vi "SW_Load_data_for_Analysis_from_TDMS.vi"(4 "Data samples to load":i64=-1, 6 "create index file? (T)":bool, 8 "error in (no error)":errorcluster, 9 "Progress bar reference":refnum<vi>, 10 "Cluster of paths input":T5, 11 "Data flow controls":T6) -> (0 "error out":errorcluster, 2 "Time to load, ms":u32, 3 "Loaded data":T1, 5 "Data loaded OK":bool, 7 "Settings loaded OK":bool)   [LabVIEW 2016]
panel:
  out "Loaded recording parameters":T2
  out "Author's name":string
  out "Stimulus presets array (loaded)":T3(array[cluster])
  out "Acquisition settings cluster out":T4
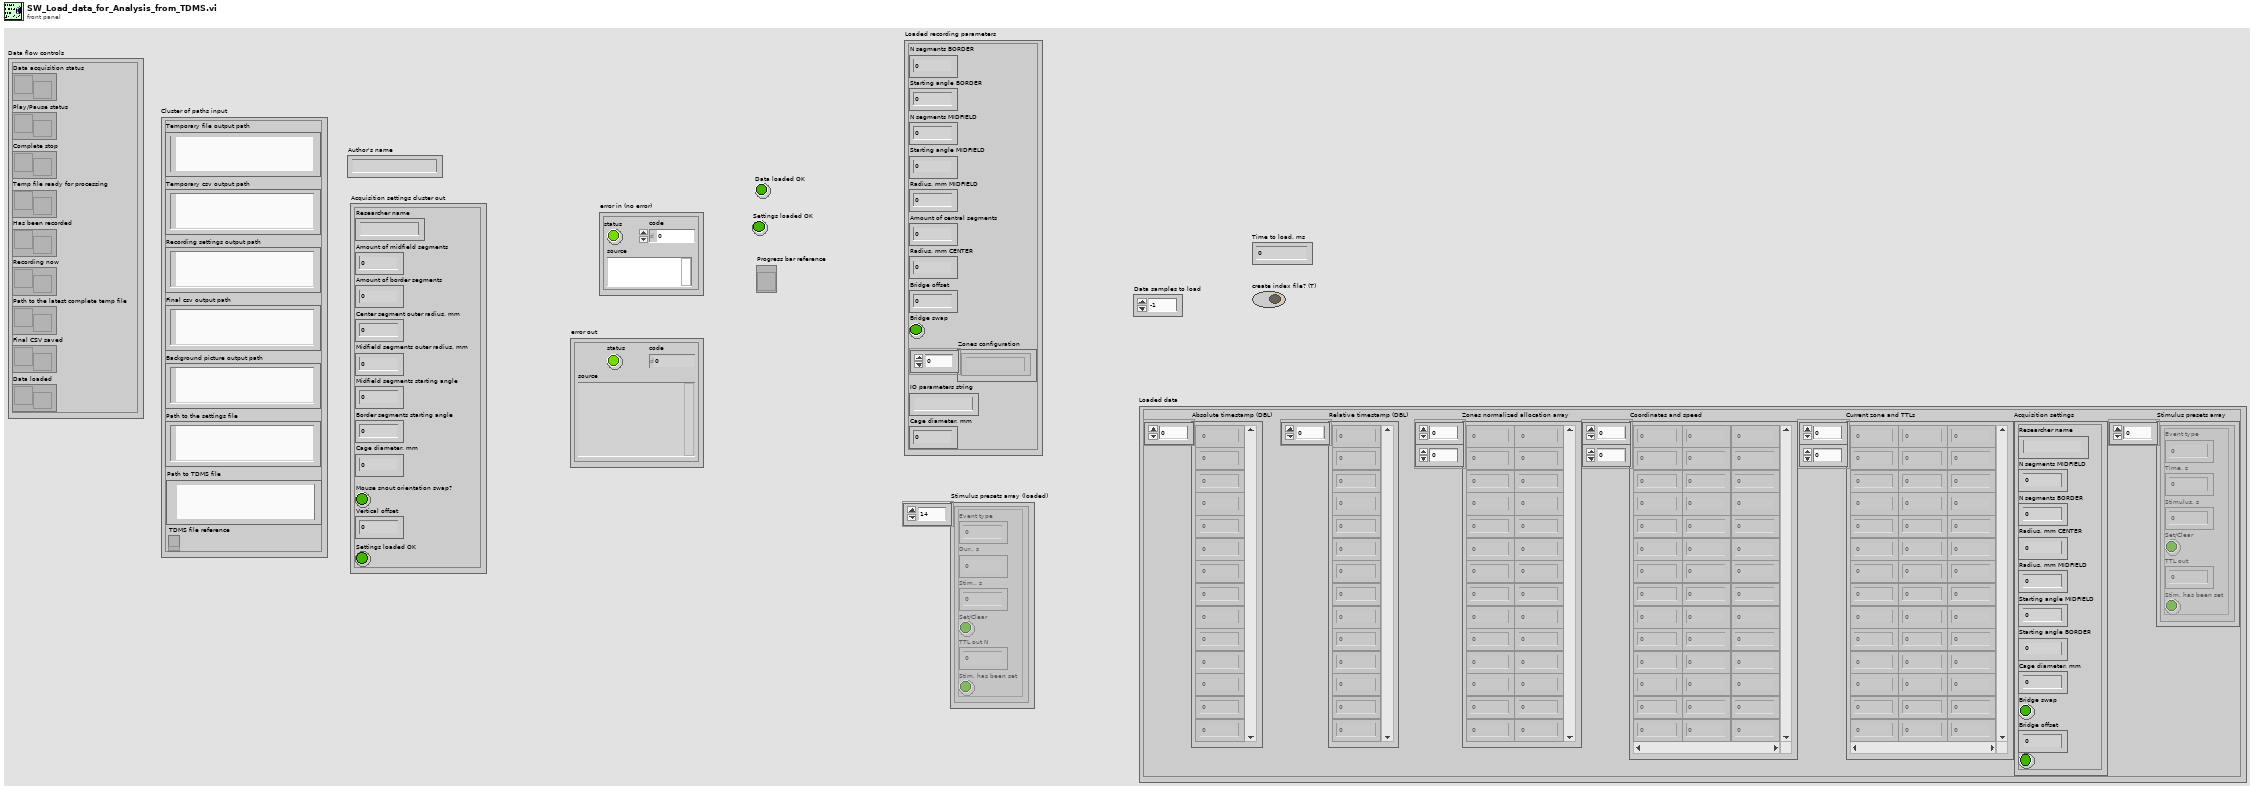
[diagram p1: front panel]
types:
  T1 = cluster{"Absolute timestamp (DBL)":dbl[], "Relative timestamp (DBL)":dbl[], "Zones normalized allocation array":dbl[][], "Coordinates and speed":dbl[][], "Current zone and TTLs":u8[][], "Acquisition settings":cluster{"Researcher name":string, "N segments MIDFIELD":u8, "N segments BORDER":u8, "Radius, mm CENTER":u16, "Radius, mm MIDFIELD":u16, "Starting angle MIDFIELD":i16, "Starting angle BORDER":i16, "Cage diameter, mm":u16, "Bridge swap":bool, "Bridge offset":sgl, "Boolean":bool}, "Stimulus presets array":cluster{"Event type":u16, "Time, s":sgl, "Stimulus, s":sgl, "Set/Clear":bool, "TTL out":u16, "Stim. has been set":bool}[]}
  T2 = cluster{"N segments BORDER":u8, "Starting angle BORDER":i16, "N segments MIDFIELD":u8, "Starting angle MIDFIELD":i16, "Radius, mm MIDFIELD":u16, "Amount of central segments":u8, "Radius, mm CENTER":u16, "Bridge offset":sgl, "Bridge swap":bool, "Zones configuration":string[], "IO parameters string":string, "Cage diameter, mm":u16}
  T3 = cluster{"Event type":u16, "Dur., s":sgl, "Stim., s":sgl, "Set/Clear":bool, "TTL out N":u16, "Stim. has been set":bool}[]
  T4 = cluster{"Researcher name":string, "Amount of midfield segments":u32, "Amount of border segments":u32, "Center segment outer radius, mm":u32, "Midfield segments outer radius, mm":u32, "Midfield segments starting angle":i32, "Border segments starting angle":i32, "Cage diameter, mm":u32, "Mouse snout orientation swap?":bool, "Vertical offset":dbl, "Settings loaded OK":bool}
  T5 = cluster{"Temporary file output path":path, "Temporary csv output path":path, "Recording settings output path":path, "Final csv output path":path, "Background picture output path":path, "Path to the settings file":path, "Path to TDMS file":path, "TDMS file reference":refnum<k34>}
  T6 = cluster{"Data acquisition status":refnum<notifier>, "Play/Pause status":refnum<notifier>, "Complete stop":refnum<notifier>, "Temp file ready for processing":refnum<notifier>, "Has been recorded":refnum<notifier>, "Recording now":refnum<notifier>, "Path to the latest complete temp file":refnum<notifier>, "Final CSV saved":refnum<notifier>, "Data loaded":refnum<notifier>}
  T7 = enum16{"big-endian, network order", "native, host order", "little-endian"}
  T8 = enum16{"open", "open or create", "create or replace", "create", "open (read-only)"}
  T9 = cluster{"Event type":u16, "Time, s":sgl, "Stimulus, s":sgl, "Set/Clear":bool, "TTL out":u16, "Stim. has been set":bool}
  T10 = cluster{string, "N segments MIDFIELD":u8, "N segments BORDER":u8, "Radius, mm CENTER":u16, "Radius, mm MIDFIELD":u16, "Starting angle MIDFIELD":i16, "Starting angle BORDER":i16, "Cage diameter, mm":u16, "Bridge swap":bool, "Bridge offset":sgl, bool}
  T11 = cluster{dbl[], dbl[], "Zones normalized allocation array":dbl[][], dbl[][], u8[][], cluster{string, "N segments MIDFIELD":u8, "N segments BORDER":u8, "Radius, mm CENTER":u16, "Radius, mm MIDFIELD":u16, "Starting angle MIDFIELD":i16, "Starting angle BORDER":i16, "Cage diameter, mm":u16, "Bridge swap":bool, "Bridge offset":sgl, bool}, cluster{"Event type":u16, "Time, s":sgl, "Stimulus, s":sgl, "Set/Clear":bool, "TTL out":u16, "Stim. has been set":bool}[]}
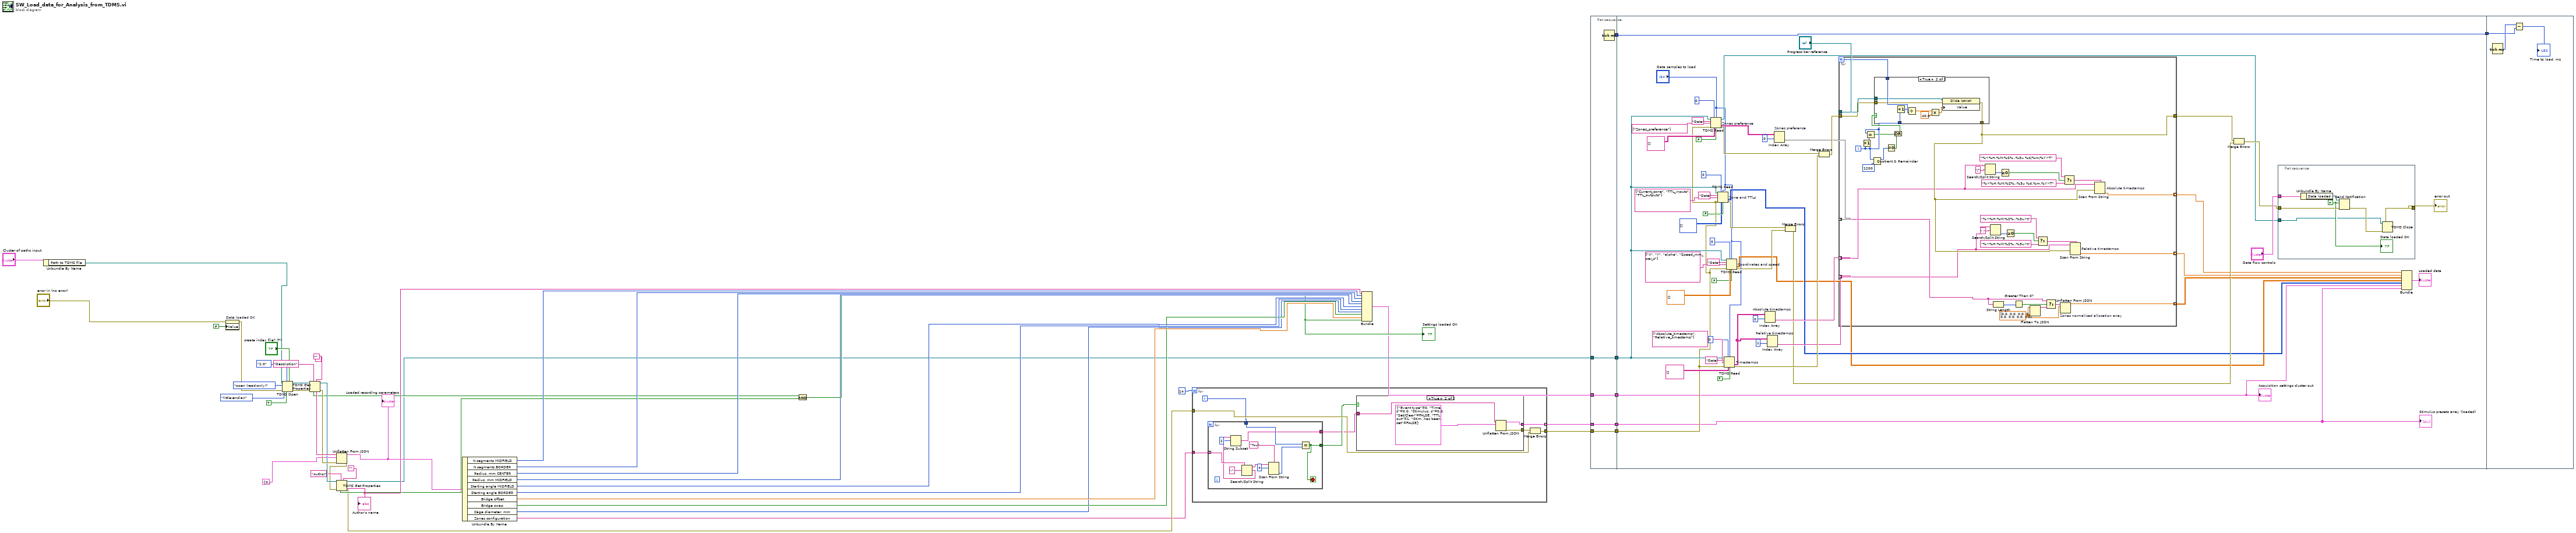
[diagram p0: block diagram]
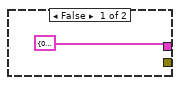
[diagram p3: hidden frame]
diagram:
  (unwired) ""
  n1 = Unbundle By Name("Cluster of paths input") -> ("Path to TDMS file"=w1:path)
  n2 = property on="Data loaded OK" class="Bool (strict)"(error in="error in (no error)", "Value"=FALSE ("Data loaded OK")) -> (error out=w9:errorcluster)  [unwired: 1 in, 1 out]
  n3 = TDMS Open(5:"create index file? (T)", 6:TRUE ("disable buffering? (T)"), 7:enum16{"1.0", "2.0"}."2.0" ("file format version (2.0)"), 8:w9, 9:T7."little-endian" ("byte order (2:little-endian)"), 10:T8."open (read-only)" ("operation (0:open)"), 11:w1) -> (0:w41:errorcluster, 3:w42:refnum<k34>)
  n4 = TDMS Get Properties(5:"", 7:"Description" ("property name"), 8:w41, 11:w42) -> (0:w37:errorcluster, 3:w36:refnum<k34>, 4:w38:string, 6:w20:bool)  [unwired: 2 in, 2 out]
  n5 = Unflatten From JSON(JSON string=w38, type and defaults=T2 {"N segments BORDER"=0, "Starting angle BORDER"=0, "N segments MIDFIELD"=0, "Starting angle MIDFIELD"=0, "Radius, mm MIDFIELD"=0, "Amount of central segments"=0, "Radius, mm CENTER"=0, "Bridge offset"=0.0, "Bridge swap"=FALSE, "Zones configuration"=[], "IO parameters string"="[12,1,1,0,0,0]", "Cage diameter, mm"=180} ("Parameters"), error in (no error)=w37) -> (value=w23:T2, error out=w33:errorcluster)  [unwired: 4 in]
  "Loaded recording parameters" <- w23
  n6 = TDMS Get Properties(5:"", 7:"Author" ("property name"), 8:w33, 11:w36) -> (0:w18:errorcluster, 3:w14:refnum<k34>, 4:w32:string, 6:w19:bool)  [unwired: 2 in, 2 out]
  "Author's name" <- w32
  n7 = Unbundle By Name(w23) -> ("N segments MIDFIELD"=w31:u8, "N segments BORDER"=w30:u8, "Radius, mm CENTER"=w29:u16, "Radius, mm MIDFIELD"=w28:u16, "Starting angle MIDFIELD"=w27:i16, "Starting angle BORDER"=w26:i16, "Bridge offset"=w25:sgl, "Bridge swap"=w24:bool, "Cage diameter, mm"=w21:u16, "Zones configuration"=w17:string[])
  n8 = And(x=w20, y=w19) -> (x .and. y?=w15:bool)
  "Settings loaded OK" <- w15
  n9 = for {
    N: 14 -> [_]
    tunnel: w18 -> [w53]
    tunnel: [w55] -> w13
    tunnel: [w56] -> w11 mode=indexing
    tunnel: w17 -> [w51]
    i -> [w52]
    n10 = for {
      tunnel: w51 -> [w67] mode=indexing
      tunnel: w52 -> [w61]
      tunnel: [w60] -> w50
      tunnel: [w59] -> w49
      stop <- w60 stop-if-true
      n11 = Search/Split String(string=w67, search string/char (-)=":") -> (substring before match=w65:string, match + rest of string=w58:string)  [unwired: 1 in, 1 out]
      n12 = String Subset(string=w58, offset (0)=2) -> (substring=w59:string)  [unwired: 1 in]
      n13 = Scan From String(format string="%u", input string=w65, initial scan location=u32 4) -> (output 1=w62:u32)  [unwired: 2 in, 3 out]
      n14 = Equal?(x=w61, y=w62) -> (x = y?=w60:bool)
    }
    n15 = case shown="True" w50 {
      tunnel: w49 -> [_ w72]
      tunnel: [T9 {"Event type"=0, "Time, s"=0.0, "Stimulus, s"=0.0, "Set/Clear"=FALSE, "TTL out"=1, "Stim. has been set"=FALSE} ("Cluster of the stimuls settings") w71] -> w56
      tunnel: [_ w70] -> w54
      frame False {
      }
      frame True {
        n16 = Unflatten From JSON(JSON string=w72, type and defaults=T9 {"Event type"=0, "Time, s"=0.0, "Stimulus, s"=0.0, "Set/Clear"=FALSE, "TTL out"=1, "Stim. has been set"=FALSE} ("Cluster of the stimuls settings")) -> (value=w71:T9, error out=w70:errorcluster)  [unwired: 5 in]
      }
    }
    n17 = Merge Errors(w54, w53) -> (w55:errorcluster)
  }
  n18 = Bundle(w32, "N segments MIDFIELD"=w31, "N segments BORDER"=w30, "Radius, mm CENTER"=w29, "Radius, mm MIDFIELD"=w28, "Starting angle MIDFIELD"=w27, "Starting angle BORDER"=w26, "Cage diameter, mm"=w21, "Bridge swap"=w24, "Bridge offset"=w25, w15) -> (w12:T10)  [unwired: 1 in]
  n19 = flat-sequence {
    tunnel: w11 -> [w74]
    tunnel: w12 -> [w75]
    tunnel: w13 -> [w76]
    tunnel: w14 -> [w77]
    tunnel: [w77] -> w7
    tunnel: [w76] -> w6
    tunnel: [w75] -> w5
    tunnel: [w74] -> w4
    tunnel: [w73] -> w3
    tunnel: w7 -> [w112]
    tunnel: w6 -> [w111]
    tunnel: w5 -> [w90]
    tunnel: w4 -> [w89]
    tunnel: w3 -> [w78]
    tunnel: [w78] -> w2
    tunnel: w2 -> [w182]
    frame #0 {
      n20 = Tick Count (ms)() -> (millisecond timer value=w73:u32)
    }
    frame #1 {
      n21 = TDMS Read "Zones preference"(0:w112, 1:i64 0 ("offset (0)"), 2:"Data samples to load", 5:"Data" ("group name in"), 7:string[] ["Zones_preference"] ("Columns Names"), 11:w111, 12:string[][] [], 13:FALSE ("return channels in file order? (F)")) -> (4:w84:refnum<k34>, 10:w97:string[][], 15:w108:errorcluster)  [unwired: 3 out]
      n22 = TDMS Read "Zone and TTLs"(0:w112, 1:i64 0 ("offset (0)"), 2:"Data samples to load", 5:"Data" ("group name in"), 7:string[] ["Current_zone", "TTL_inputs", "TTL_outputs"] ("Columns Names"), 11:w111, 12:u8[][] [], 13:FALSE ("return channels in file order? (F)")) -> (10:w87:u8[][], 15:w106:errorcluster)  [unwired: 4 out]
      n23 = TDMS Read "Timestamps"(0:w112, 1:i64 0 ("offset (0)"), 2:"Data samples to load", 5:"Data" ("group name in"), 7:string[] ["Absolute_timestamp", "Relative_timestamp"] ("Columns Names"), 11:w111, 12:string[][] [], 13:FALSE ("return channels in file order? (F)")) -> (10:w101:string[][], 15:w107:errorcluster)  [unwired: 4 out]
      n24 = TDMS Read "Coordinates and speed"(0:w112, 1:i64 0 ("offset (0)"), 2:"Data samples to load", 5:"Data" ("group name in"), 7:string[] ["X", "Y", "alpha", "Speed_mm_per_s"] ("Columns Names"), 11:w111, 12:dbl[][] [], 13:FALSE ("return channels in file order? (F)")) -> (10:w86:dbl[][], 15:w95:errorcluster)  [unwired: 4 out]
      n25 = Index Array "Absolute timestamps"(array=w101, index (row)=0) -> (element=w100:string[])  [unwired: 1 in]
      n26 = Index Array "Relative timestamps"(array=w101, index (row)=1) -> (element=w99:string[])  [unwired: 1 in]
      n27 = Index Array "Zones preference"(array=w97, index (row)=0) -> (element=w96:string[])  [unwired: 1 in]
      n28 = Merge Errors(w106, w95) -> (w94:errorcluster)
      n29 = Merge Errors(w108, w107) -> (w109:errorcluster)
      n30 = for {
        N -> [w163]
        tunnel: w109 -> [w161]
        tunnel: [w148] -> w105
        tunnel: "Progress bar reference" -> [w162]
        tunnel: w100 -> [w140] mode=indexing
        tunnel: w99 -> [w138] mode=indexing
        tunnel: w96 -> [w142] mode=indexing
        tunnel: [w141] -> w91 mode=indexing
        tunnel: [w139] -> w93 mode=indexing
        tunnel: [w137] -> w92 mode=indexing
        i -> [w132]
        w143 = dbl[] [0.0, 0.0, 0.0, 0.0, 0.0, 0.0, 0.0, 0.0, 0.0] ("Zones normalized allocation array")
        n31 = Increment(x=w132) -> (x+1=w130:i32)
        n32 = Equal?(x=w132, y=w130) -> (x = y?=w131:bool)
        n33 = Quotient & Remainder(x=w132, y=1200) -> (x-y*floor(x/y)=w135:i32)  [unwired: 1 out]
        n34 = Equal To 0?(x=w135) -> (x = 0?=w134:bool)
        n35 = Or(x=w131, y=w134) -> (x .or. y?=w133:bool)
        n36 = case shown="True" w133 {
          tunnel: w132 -> [_ w173]
          tunnel: w163 -> [_ w172]
          tunnel: w162 -> [_ w171]
          tunnel: w161 -> [w164 w170]
          tunnel: [w164 w169] -> w148
          frame False {
          }
          frame True {
            n37 = Increment(x=w173) -> (x+1=w166:i32)
            n38 = Divide(x=w166, y=w172) -> (x/y=w168:dbl)
            n39 = Multiply(x=w168, y=40.0) -> (x*y=w165:dbl)
            n40 = property on="Property Node" class="Slide (strict)"(reference=w171, error in=w170, "Value"=w165) -> (error out=w169:errorcluster)  [unwired: 1 out]
          }
        }
        n41 = Search/Split String(string=w140, search string/char (-)="/") -> (offset of match=w156:i32)  [unwired: 1 in, 2 out]
        n42 = Search/Split String(string=w138, search string/char (-)=".") -> (offset of match=w152:i32)  [unwired: 1 in, 2 out]
        n43 = String Length(string=w142) -> (length=w147:i32)
        n44 = Greater Or Equal To 0?(x=w156) -> (x >= 0?=w155:bool)
        n45 = Greater Or Equal To 0?(x=w152) -> (x >= 0?=w149:bool)
        n46 = Greater Than 0?(x=w147) -> (x > 0?=w146:bool)
        n47 = Flatten To JSON(anything=w143) -> (JSON string=w144:string)  [unwired: 2 in, 1 out]
        n48 = Select(t="%<%H:%M:%S%.;%3u>t" ("format string"), s=w149, f="%<%H:%M:%S%,;%3u>t" ("format string")) -> (s? t:f=w154:string)
        n49 = Select(t=w142, s=w146, f=w144) -> (s? t:f=w145:string)
        n50 = Unflatten From JSON "Zones normalized allocation array"(JSON string=w145, type and defaults=w143) -> (value=w141:dbl[])  [unwired: 5 in, 1 out]
        n51 = Select(t="%<%H:%M:%S%.;%3u %d/%m/%Y>T" ("format string"), s=w155, f="%<%H:%M:%S%,;%3u %d.%m.%Y>T" ("format string")) -> (s? t:f=w158:string)
        n52 = Scan From String "Relative timestamps"(format string=w154, input string=w138, error in=w148) -> (output 1=w137:dbl)  [unwired: 2 in, 3 out]
        n53 = Scan From String "Absolute timestamps"(format string=w158, input string=w140, error in=w148) -> (output 1=w139:dbl)  [unwired: 2 in, 3 out]
      }
      n54 = Merge Errors(w105, w94) -> (w104:errorcluster)
      n55 = flat-sequence {
        tunnel: "Data flow controls" -> [w180]
        tunnel: [w176] -> w85
        tunnel: w104 -> [w179]
        tunnel: w84 -> [w175]
        frame #0 {
          w178 = TRUE ("notification")
          n56 = Unbundle By Name(w180) -> ("Data loaded"=w174:refnum<notifier>)
          n57 = Send Notification(notification=w178, notifier=w174, error in (no error)=w179) -> (error out=w177:errorcluster)  [unwired: 1 out]
          n58 = TDMS Close(8:w177, 11:w175) -> (0:w176:errorcluster)  [unwired: 1 out]
          "Data loaded OK" <- w178
        }
      }
      n59 = Bundle(w93, w92, "Zones normalized allocation array"=w91, w86, w87, w90, w89) -> (→"Loaded data":T11)  [unwired: 1 in]
      "error out" <- w85
      "Acquisition settings cluster out" <- w90
      "Stimulus presets array (loaded)" <- w89
    }
    frame #2 {
      n60 = Tick Count (ms)() -> (millisecond timer value=w183:u32)
      n61 = Subtract(x=w183, y=w182) -> (x-y=→"Time to load, ms":u32)
    }
  }
